vi "mtg - get seconds in the hour.vi"(8 "error in (no error)":errorcluster) -> (2 "seconds into the hour":i32)   [LabVIEW 2025]
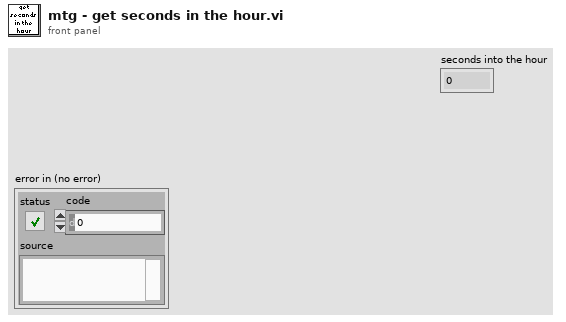
[diagram p1: front panel]
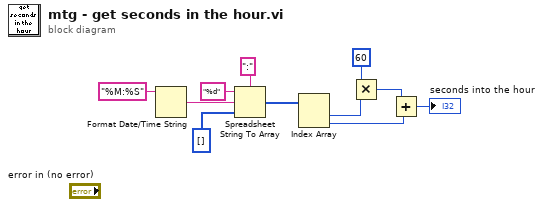
[diagram p0: block diagram]
diagram:
  n1 = Format Date/Time String(time format string (%c)="%M:%S") -> (date/time string=w10:string)  [unwired: 2 in]
  n2 = Spreadsheet String To Array(delimiter (Tab)=":", format string="%d", spreadsheet string=w10, array type (2D Dbl)=i32[] []) -> (array=w6:i32[])
  n3 = Index Array(array=w6) -> (element #1=w5:i32, element #2=w2:i32)  [unwired: 2 in]
  n4 = Multiply(x=60, y=w5) -> (x*y=w3:i32)
  n5 = Add(x=w3, y=w2) -> (x+y=→"seconds into the hour":i32)
